vi "XMLStatusMessage.vi"(8 "error in (no error)":errorcluster caption="错误输入（无错误）") -> (0 "error out":errorcluster caption="错误输出", 3 "连接的字符串":string)   [LabVIEW 2018]
uses:
  Subvi/Global.vi
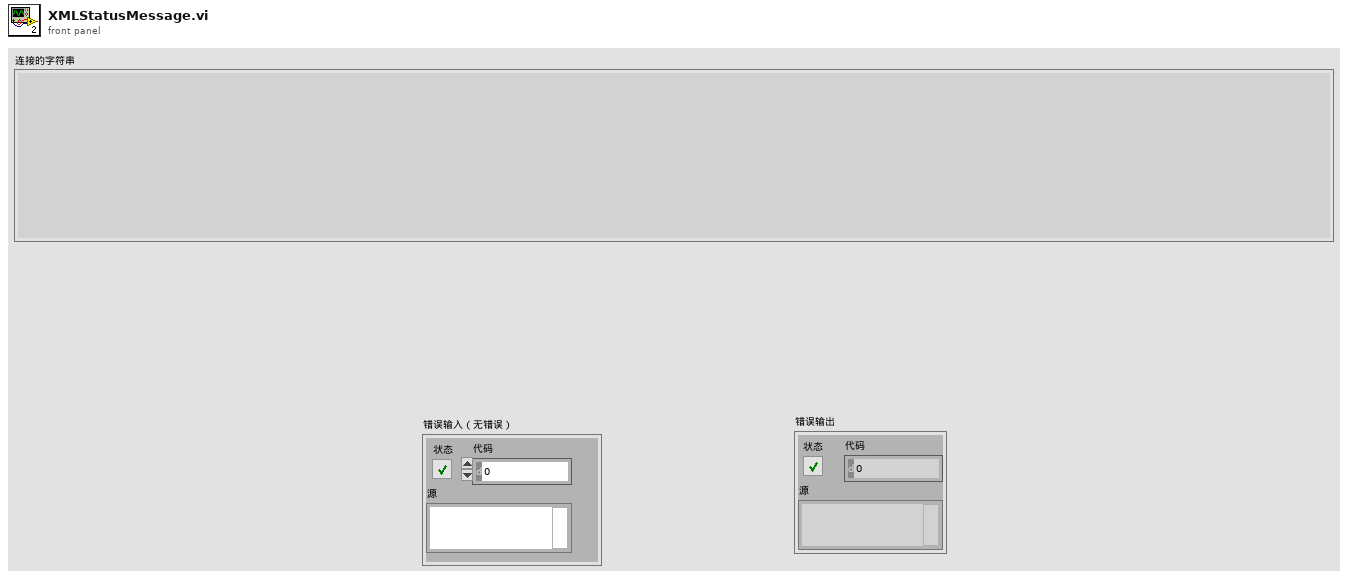
[diagram p1: front panel]
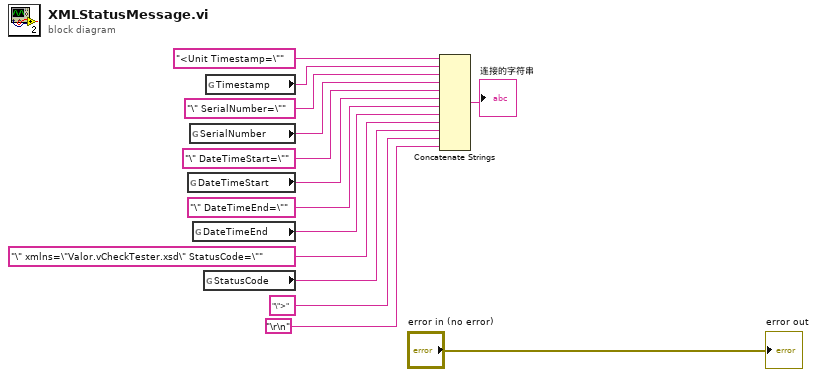
[diagram p0: block diagram]
diagram:
  n1 = global read "Global.vi" "DateTimeStart"() -> (w9:string)
  n2 = global read "Global.vi" "SerialNumber"() -> (w11:string)
  n3 = global read "Global.vi" "DateTimeEnd"() -> (w7:string)
  n4 = global read "Global.vi" "StatusCode"() -> (w5:string)
  n5 = global read "Global.vi" "Timestamp"() -> (w13:string)
  n6 = Concatenate Strings("<Unit Timestamp=\"", w13, "\" SerialNumber=\"", w11, "\" DateTimeStart=\"", w9, "\" DateTimeEnd=\"", w7, "\" xmlns=\"Valor.vCheckTester.xsd\" StatusCode=\"", w5, "\">", "\r\n") -> (→"连接的字符串":string)
  "error out" <- "error in (no error)"
